vi "SpinnySetPos.vi"(0 "Arduino Resource":T1={"VISA resource"="", "Board Type"=enum."Uno", "Connection Type"=enum."USB / Serial", "Bytes Per Packet (15)"=15}, 1 "stepper #":u8=1, 3 "position":i32, 5 "error in":errorcluster) -> (14 "Arduino Resource Out":T1={"VISA resource"="", "Board Type"=enum."Uno", "Connection Type"=enum."USB / Serial", "Bytes Per Packet (15)"=15}, 15 "PositionBotBot":i32, 16 "Position Bot":i32, 19 "error out":errorcluster)   [LabVIEW 2014]
doc: "return current position of nth stepper in steps"
uses:
  <vilib>/LabVIEW Interface for Arduino/Type Defs/Arduino Resource.ctl
  <vilib>/LabVIEW Interface for Arduino/Type Defs/Board Type.ctl
  <vilib>/LabVIEW Interface for Arduino/LabVIEW Interface for Arduino.lvlib
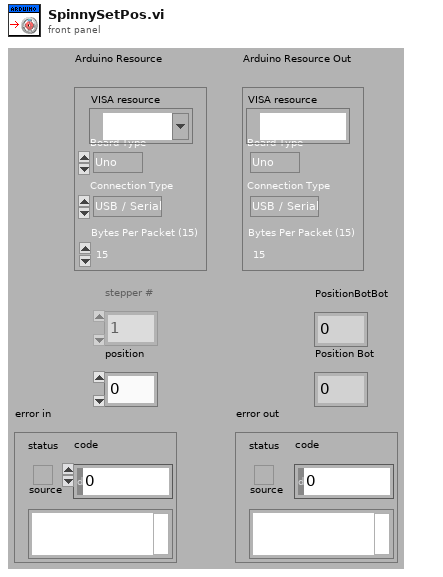
[diagram p1: front panel]
types:
  T1 = typedef "LabVIEW Interface for Arduino.lvlib/Arduino Resource.ctl" = cluster{"VISA resource":refnum<visa-resource-name>, "Board Type":T2, "Connection Type":enum8{"USB / Serial"}, "Bytes Per Packet (15)":u8}
  T2 = typedef "LabVIEW Interface for Arduino.lvlib/Board Type.ctl" = enum16{"Uno", "Dimuelanove w/Atmega 328", "Mega 2560"}
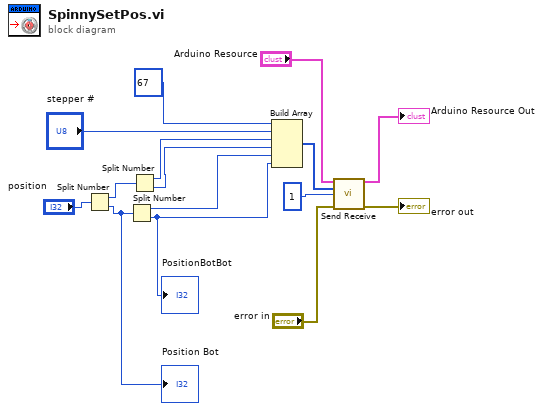
[diagram p0: block diagram]
diagram:
  n1 = Split Number(x="position") -> (hi(x)=w3:u16, lo(x)=w4:u16)
  "Position Bot" <- w4
  n2 = Split Number(x=w4) -> (hi(x)=w2:u8, lo(x)=w1:u8)
  "PositionBotBot" <- w1
  n3 = Split Number(x=w3) -> (hi(x)=w7:u8, lo(x)=w6:u8)
  n4 = Build Array(u8 67, "stepper #", w7, w6, w2, w1) -> (w9:u8[])
  n5 = call <vilib>:"Send Receive.vi"("Arduino Resource"="Arduino Resource", "Data"=w9, "Bytes To Read (0)"=u8 1, "error in"="error in") -> ("Arduino Resource"=→"Arduino Resource Out":T1, "error out"=→"error out":errorcluster)  [unwired: 9 in, 1 out]
